vi "Init IPC.vi"(8 "error in (no error)":errorcluster, 11 "TCPMessaging in":refnum<class "TCPMessaging.lvclass">) -> (0 "error out":errorcluster, 3 "TCPMessaging out":refnum<class "TCPMessaging.lvclass">)   [LabVIEW 2020, in "Vecto.lvlib" / "TCPMessaging.lvclass"]
uses:
  TCPMessaging.lvclass
  Send Message Data.ctl
  <vilib>/IlluminatedG/IG Promises/Promises/Promise/Promise.lvclass
  proto/TcpPayload/Data.ctl
  TCPConnectionHandler/TCPConnectionHandler.lvclass
  TCPMessageHandler/TCPMessageHandler.lvclass
  Request Registration.ctl
  TCPMessaging.lvclass/TCPMessaging.ctl
  TX Payload.ctl
  Client Action Data.ctl
  Client Action.ctl
  Client Info.ctl
  proto/TcpClientHello/Data.ctl
  proto/TcpClientHello/TcpClientHello.lvlib
  Vecto.lvlib
  proto/TcpPayload/TcpPayload.lvlib
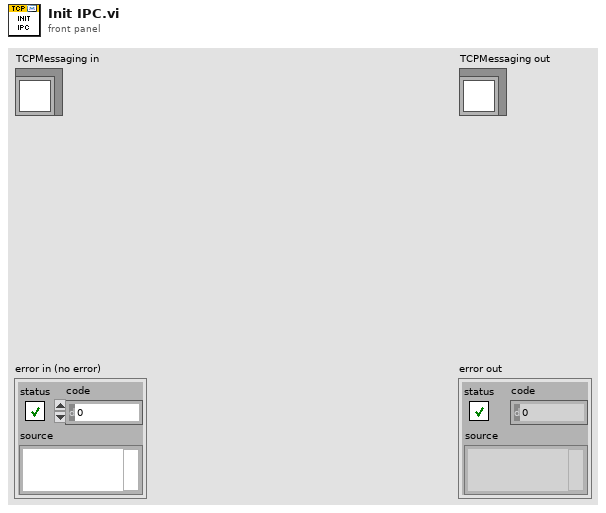
[diagram p1: front panel]
types:
  T1 = typedef "Vecto.lvlib/TCPMessaging.lvclass/Request Registration.ctl" = cluster{"Sequence":u32, "Reply Promise":refnum<class "Promise.lvclass">, "Reply Deadline":dbl}
  T2 = typedef "TcpPayload.lvlib/Data.ctl" = cluster{"target_node":u32, "target_task":u32, "source_id":u32, "sequence":u32, "timestamp":u64, "type_id":u32, "payload":u8[]}
  T3 = typedef "Vecto.lvlib/Send Message Data.ctl" = cluster{"TcpPayload":T2, "Register Reply":bool, "Reply Promise":refnum<class "Promise.lvclass">, "Reply Deadline":dbl}
  T4 = typedef "Vecto.lvlib/TCPMessaging.lvclass/TCP Mode.ctl" = enum16{"Client", "Server"}
  T5 = typedef "Vecto.lvlib/Client Info.ctl" = cluster{"TcpClientHello":T6, "Remote Address":string, "Remote Port":u16}
  T6 = typedef "TcpClientHello.lvlib/Data.ctl" = cluster{"node_id":u32, "system":string, "cluster":string, "node_name":string, "app_version":string, "config_version":string}
  T7 = typedef "Vecto.lvlib/TCPMessaging.lvclass/Client Action Data.ctl" = cluster{"Client Action":T8, "Client Info":T5, "TCP":refnum<k5>, "TX Q":refnum<queue>}
  T8 = typedef "Vecto.lvlib/TCPMessaging.lvclass/Client Action.ctl" = enum16{"Connect", "Ready", "Disconnect"}
  T9 = typedef "Vecto.lvlib/TX Payload.ctl" = cluster{"Target ID":u32, "Payload":string}
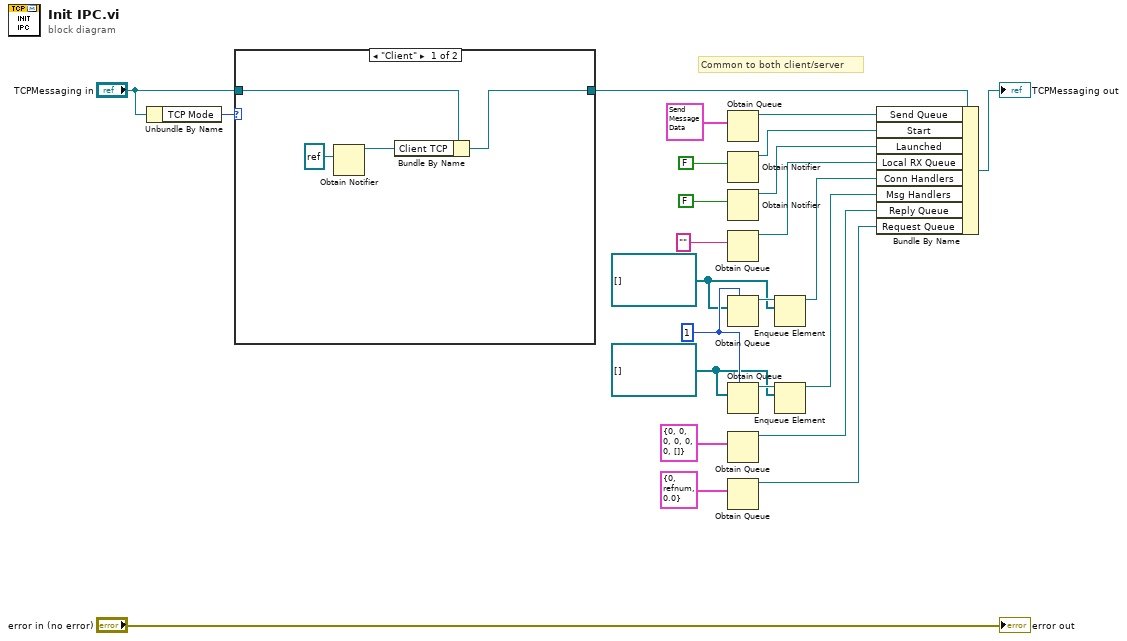
[diagram p0: block diagram]
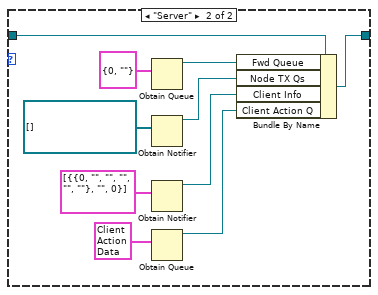
[diagram p2: hidden frame]
diagram:
  w10 = 1 ("max queue size (-1, unlimited)")
  w7 = refnum<class "TCPMessageHandler.lvclass">[] []
  w9 = refnum<class "TCPConnectionHandler.lvclass">[] [] ("Array")
  # "Common to both client/server"
  n1 = Unbundle By Name("TCPMessaging in") -> ("TCP Mode"=w22:T4)
  n2 = case shown="\"Client\"" w22 {
    tunnel: "TCPMessaging in" -> [w27 w38]
    tunnel: [w28 w36] -> w15
    frame "Client" {
      n3 = Obtain Notifier(notification data type=refnum<k5> refnum ("connection ID")) -> (notifier out=w25:refnum<notifier>)  [unwired: 3 in, 2 out]
      n4 = Bundle By Name(cluster=w27, "Client TCP"=w25) -> (w28:refnum<class "TCPMessaging.lvclass">)
    }
    frame "Server" {
      n5 = Obtain Queue(element data type=T9 {"Target ID"=0, "Payload"=""} ("TX Payload")) -> (queue out=w34:refnum<queue>)  [unwired: 4 in, 2 out]
      n6 = Obtain Notifier(notification data type=refnum<queue>[] [] ("queue out")) -> (notifier out=w32:refnum<notifier>)  [unwired: 3 in, 2 out]
      n7 = Obtain Notifier(notification data type=T5[] [{"TcpClientHello"={"node_id"=0, "system"="", "cluster"="", "node_name"="", "app_version"="", "config_version"=""}, "Remote Address"="", "Remote Port"=0}]) -> (notifier out=w33:refnum<notifier>)  [unwired: 3 in, 2 out]
      n8 = Obtain Queue(element data type=T7 {"Client Action"=enum."Disconnect", "Client Info"={"TcpClientHello"={"node_id"=0, "system"="", "cluster"="", "node_name"="", "app_version"="", "config_version"=""}, "Remote Address"="", "Remote Port"=0}, "TCP"=refnum, "TX Q"=refnum} ("Client Action Data")) -> (queue out=w30:refnum<queue>)  [unwired: 4 in, 2 out]
      n9 = Bundle By Name(cluster=w38, "Fwd Queue"=w34, "Node TX Qs"=w32, "Client Info"=w33, "Client Action Q"=w30) -> (w36:refnum<class "TCPMessaging.lvclass">)
    }
  }
  n10 = Obtain Queue(element data type=T3 {"TcpPayload"={"target_node"=0, "target_task"=0, "source_id"=0, "sequence"=0, "timestamp"=0, "type_id"=0, "payload"=[]}, "Register Reply"=FALSE, "Reply Promise"=refnum, "Reply Deadline"=0.0} ("Send Message Data")) -> (queue out=w20:refnum<queue>)  [unwired: 4 in, 2 out]
  n11 = Obtain Notifier(notification data type=FALSE) -> (notifier out=w21:refnum<notifier>)  [unwired: 3 in, 2 out]
  n12 = Obtain Notifier(notification data type=FALSE) -> (notifier out=w16:refnum<notifier>)  [unwired: 3 in, 2 out]
  n13 = Obtain Queue(element data type="") -> (queue out=w12:refnum<queue>)  [unwired: 4 in, 2 out]
  n14 = Obtain Queue(max queue size (-1, unlimited)=w10, element data type=w9) -> (queue out=w11:refnum<queue>)  [unwired: 3 in, 2 out]
  n15 = Obtain Queue(max queue size (-1, unlimited)=w10, element data type=w7) -> (queue out=w8:refnum<queue>)  [unwired: 3 in, 2 out]
  n16 = Obtain Queue(element data type=T2 {"target_node"=0, "target_task"=0, "source_id"=0, "sequence"=0, "timestamp"=0, "type_id"=0, "payload"=[]} ("TcpPayload")) -> (queue out=w3:refnum<queue>)  [unwired: 4 in, 2 out]
  n17 = Obtain Queue(element data type=T1 {"Sequence"=0, "Reply Promise"=refnum, "Reply Deadline"=0.0} ("Request Registration")) -> (queue out=w1:refnum<queue>)  [unwired: 4 in, 2 out]
  n18 = Enqueue Element(queue=w11, element=w9) -> (queue out=w6:refnum<queue>)  [unwired: 2 in, 2 out]
  n19 = Enqueue Element(queue=w8, element=w7) -> (queue out=w5:refnum<queue>)  [unwired: 2 in, 2 out]
  n20 = Bundle By Name(cluster=w15, "Send Queue"=w20, "Start"=w21, "Launched"=w16, "Local RX Queue"=w12, "Conn Handlers"=w6, "Msg Handlers"=w5, "Reply Queue"=w3, "Request Queue"=w1) -> (→"TCPMessaging out":refnum<class "TCPMessaging.lvclass">)
  "error out" <- "error in (no error)"
